vi "3) Programa Adquisición Medidas.vi"() -> ()   [LabVIEW 2014]
panel:
  in  "Selección de canal":u16(ring) items=["Canal 1", "Canal 2", "Matemático"]
  in  "stop":bool
  out "error out":errorcluster
  out "VISA resource name out":refnum<visa-resource-name>
  out "Medidas":string
  in  "error in (no error)":errorcluster
  in  "VISA resource name":refnum<visa-resource-name>
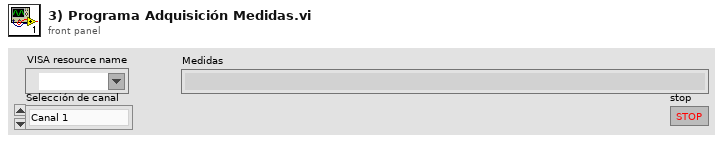
[diagram p1: front panel]
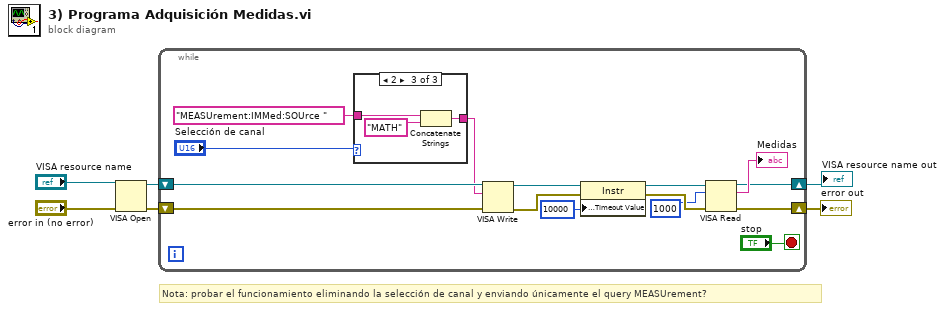
[diagram p0: block diagram]
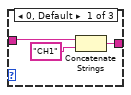
[diagram p2: hidden frame]
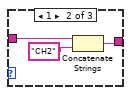
[diagram p3: hidden frame]
diagram:
  # "Nota: probar el funcionamiento eliminando la selección de canal y enviando únicamente el query MEASUrement?"
  n1 = VISA Open(error in (no error)="error in (no error)", VISA resource name="VISA resource name") -> (VISA resource name=w4:refnum<visa-resource-name>, error out=w3:errorcluster)  [unwired: 3 in]
  n2 = while {
    shift-right: [w13] -> w2
    shift-left: w4 -> [w21]
    shift-right: [w12] -> w1
    shift-left: w3 -> [w20]
    stop <- "stop" stop-if-true
    n3 = case shown="2" "Selección de canal" {
      tunnel: "MEASUrement:IMMed:SOUrce " -> [w23 w27 w30]
      tunnel: [w22 w25 w28] -> w9
      frame 0, Default {
        n4 = Concatenate Strings(w23, "CH1") -> (w22:string)
      }
      frame 1 {
        n5 = Concatenate Strings(w27, "CH2") -> (w25:string)
      }
      frame 2 {
        n6 = Concatenate Strings(w30, "MATH") -> (w28:string)
      }
    }
    n7 = VISA Write(VISA resource name=w21, write buffer=w9, error in (no error)=w20) -> (VISA resource name out=w18:refnum<visa-resource-name>, error out=w10:errorcluster)  [unwired: 1 out]
    n8 = property class="Instr"(reference=w18, error in=w10, "General Settings:Timeout Value"=u32 10000) -> (reference out=w16:refnum<visa-resource-name>, error out=w17:errorcluster)
    n9 = VISA Read(VISA resource name=w16, byte count=u32 1000, error in (no error)=w17) -> (VISA resource name out=w13:refnum<visa-resource-name>, read buffer=→"Medidas":string, error out=w12:errorcluster)  [unwired: 1 out]
  }
  "VISA resource name out" <- w2
  "error out" <- w1
